vi "Main UI.vi"() -> ()   [LabVIEW 2020, in "App.lvlib" / "MazeUI.lvclass"]
uses:
  MazeUI.lvclass
  build/ppl/maze.lvlibp/Maze/Maze.lvclass
  build/ppl/maze.lvlibp/Mouse/Mouse.lvclass
  build/ppl/maze.lvlibp/Direction.ctl
  <vilib>/Platform/browser.llb/Open URL in Default Browser (string).vi
  build/ppl/maze.lvlibp
  MazeFileIO/MazeFileIO.lvclass
  build/ppl/maze.lvlibp/MazeGen/MazeGen.lvclass
panel:
  in  "Forums":bool
  in  "Configure Mouse":bool
  out "Mouse Name":string="Demo Mouse"
  in  "Run Speed":i32(slide)=100 scale=500.0..0.5
  out "Stepping":bool
  in  "Reset":bool
  in  "Step":bool
  out "Path":picture
  out "Walls":picture
  out "Actions":i32
  out "Mouse":refnum<class "Mouse.lvclass">
  in  "Stop":bool
  out "Running":bool
  out "Maze":refnum<class "Maze.lvclass">
  in  "Save":bool
  in  "Random":bool
  out "Maze":string
  in  "Load Maze":bool
  out "Status":string
  out "Mouse Author":string="Demo Mouse"
  in  "Load Mouse":bool
  in  "Start":bool
  out "Display":picture
  # "Maze Challenge"
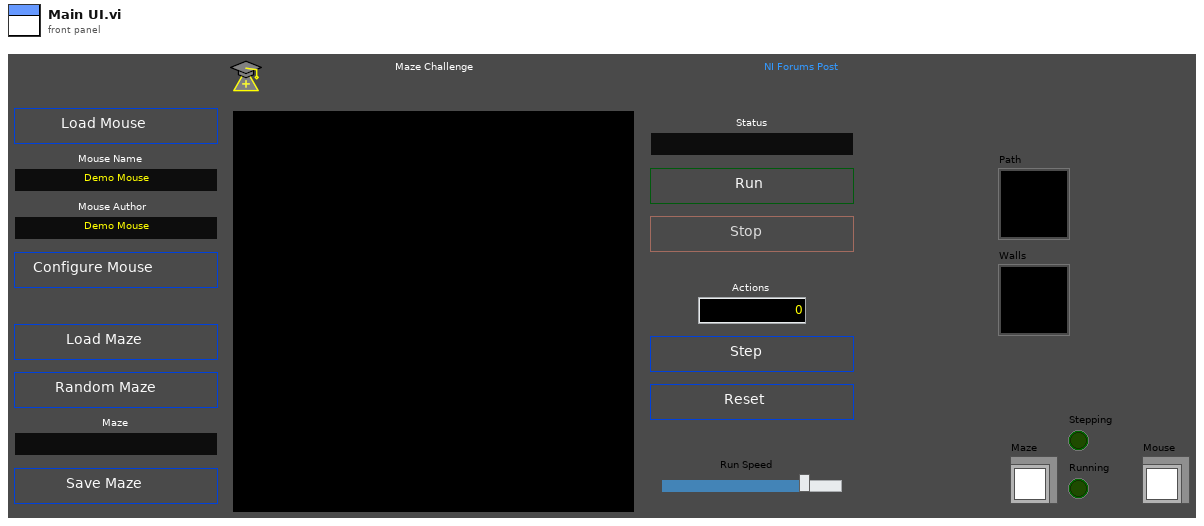
[diagram p1: front panel]
types:
  T1 = enum8{"Enabled", "Disabled", "Disabled and Grayed Out"}
  T2 = typedef "maze.lvlibp/Direction.ctl" = enum8{"East", "North", "West", "South"}
  T3 = typedef "maze.lvlibp/Position.ctl" = cluster{"S":i32, "E":i32}
  T4 = enum32{"invalid app kind", "Development System", "Run Time System", "Student Edition", "Embedded LabVIEW", "Evaluation", "Custom"}
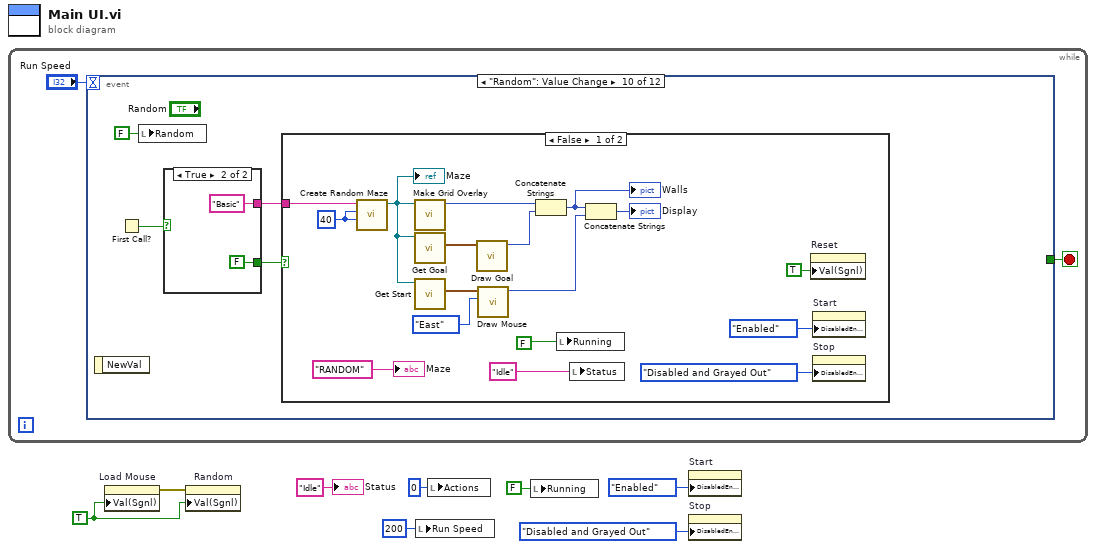
[diagram p0: block diagram]
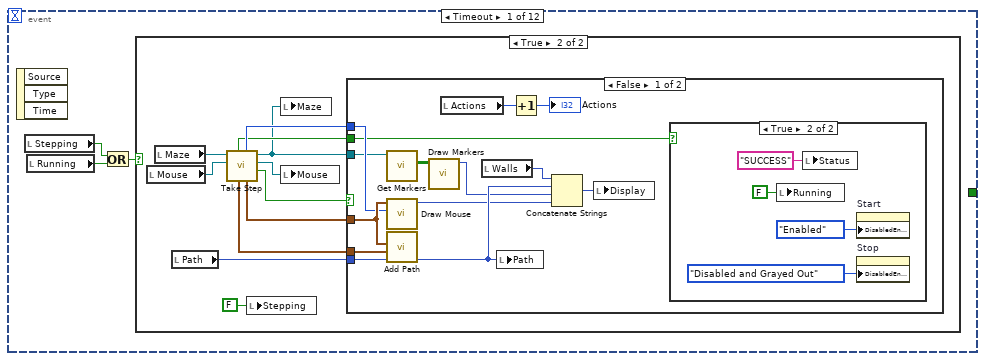
[diagram p2: hidden frame]
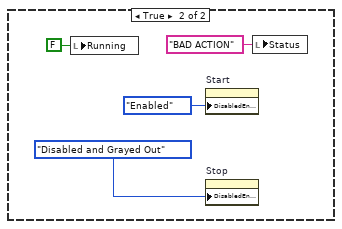
[diagram p5: hidden frame]
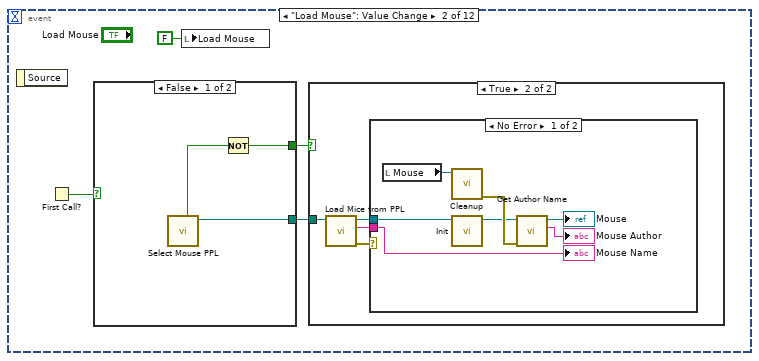
[diagram p6: hidden frame]
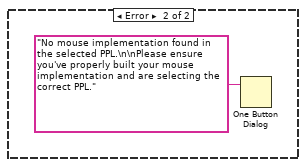
[diagram p8: hidden frame]
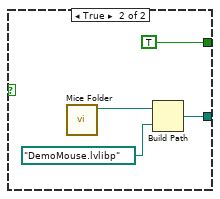
[diagram p9: hidden frame]
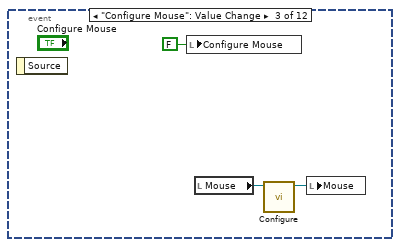
[diagram p10: hidden frame]
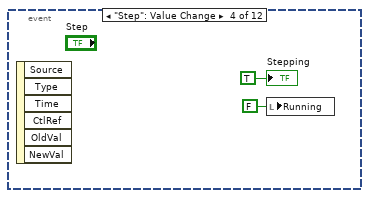
[diagram p11: hidden frame]
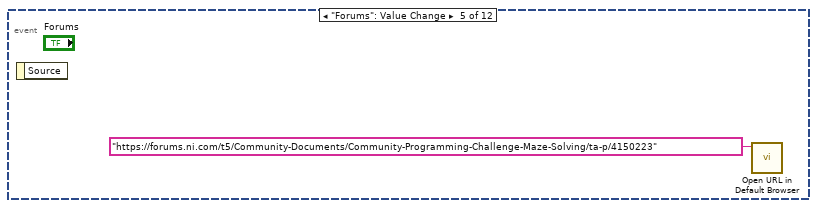
[diagram p12: hidden frame]
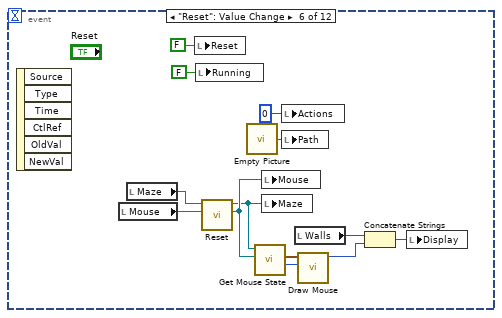
[diagram p13: hidden frame]
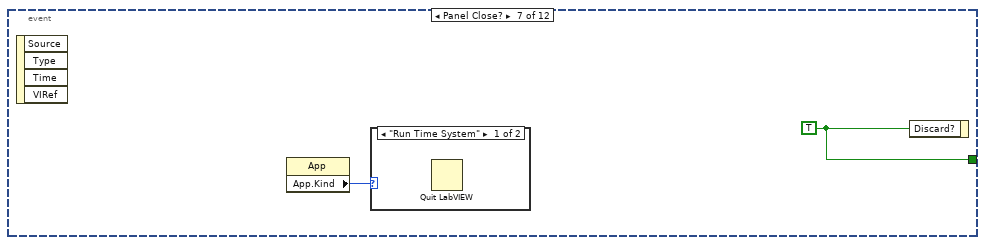
[diagram p14: hidden frame]
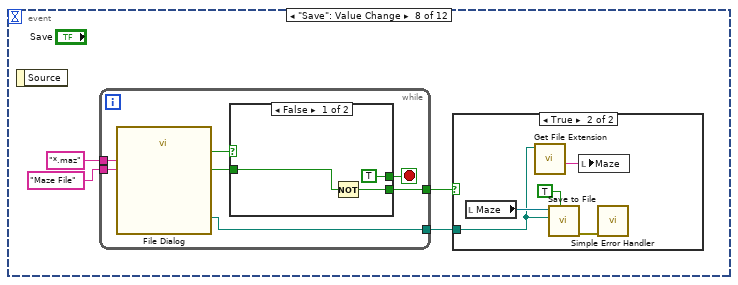
[diagram p16: hidden frame]
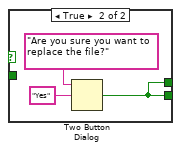
[diagram p18: hidden frame]
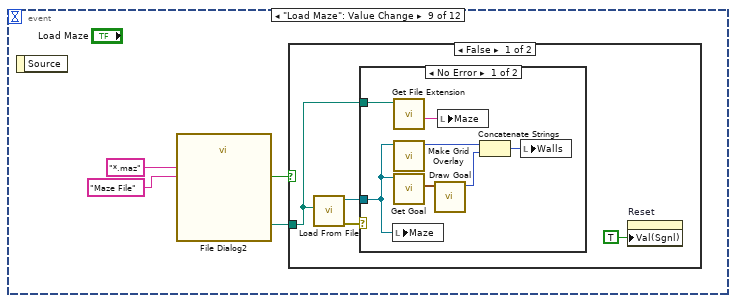
[diagram p19: hidden frame]
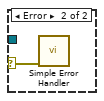
[diagram p20: hidden frame]
diagram:
  w2 = TRUE ("Value (Signaling)")
  n1 = while {
    stop <- w10 stop-if-true
    n2 = event shown="[9] \"Random\": Value Change" {
      selector: _ -> [_ _ _ _ _ _ _ _ _ _ _ _]
      dyn-events: _ -> [_ _ _ _ _ _ _ _ _ _ _ _]
      timeout: "Run Speed" -> [_ _ _ _ _ _ _ _ _ _ _ _]
      tunnel: [_ _ _ _ _ _ w90 _ _ _ _ _] -> w10
      event Timeout {
        n3 = event-data() -> ()  [unwired: 1 in, 3 out]
        n4 = local read "Stepping"() -> (w11:bool)
        n5 = local read "Running"() -> (w13:bool)
        n6 = Or(x=w11, y=w13) -> (x .or. y?=w12:bool)
        n7 = case shown="True" w12 {
          frame False {
          }
          frame True {
            n8 = local read "Mouse"() -> (w16:refnum<class "Mouse.lvclass">)
            n9 = local read "Maze"() -> (w24:refnum<class "Maze.lvclass">)
            n10 = local read "Path"() -> (w19:picture)
            n11 = call "Take Step.vi"("Mouse In"=w16, "Maze in"=w24) -> ("Bad Action?"=w23:bool, "Mouse"=w17:refnum<class "Mouse.lvclass">, "Maze"=w14:refnum<class "Maze.lvclass">, "New Position"=w21:T3, "Direction"=w22:T2, "Old Position"=w20:T3, "Goal?"=w15:bool)  [unwired: 2 in, 1 out]
            n12 = local write "Stepping"(FALSE ("Stepping")) -> ()
            n13 = local write "Maze"(w14) -> ()
            n14 = local write "Mouse"(w17) -> ()
            n15 = case shown="False" w23 {
              tunnel: w22 -> [w30 _]
              tunnel: w21 -> [w31 _]
              tunnel: w20 -> [w37 _]
              tunnel: w19 -> [w38 _]
              tunnel: w15 -> [w29 _]
              tunnel: w14 -> [w27 _]
              frame False {
                n16 = call "Get Markers.vi"("Maze in"=w27) -> ("Markers"=w26:bool[][])  [unwired: 8 in, 2 out]
                n17 = call "Draw Mouse.vi"("Direction"=w30, "Position"=w31) -> ("Picture"=w28:picture)  [unwired: 9 in]
                n18 = call "Add Path.vi"("Path In"=w38, "Old Position"=w37, "New Position"=w31) -> ("Path"=w35:picture)  [unwired: 8 in]
                n19 = call "Draw Markers.vi"("Markers"=w26) -> ("Picture"=w25:picture)  [unwired: 10 in]
                n20 = local read "Actions"() -> (w33:i32)
                n21 = local read "Walls"() -> (w36:picture)
                n22 = local write "Path"(w35) -> ()
                n23 = Increment(x=w33) -> (x+1=→"Actions":i32)
                n24 = Concatenate Strings(w36, w35, w25, w28) -> (w34:picture)
                n25 = local write "Display"(w34) -> ()
                n26 = case shown="True" w29 {
                  frame False {
                  }
                  frame True {
                    n27 = local write "Running"(FALSE ("Running")) -> ()
                    n28 = local write "Status"("SUCCESS" ("Status")) -> ()
                    n29 = property on="Start" class="Bool"("DisabledEnum"=T1."Enabled" ("Disabled")) -> ()  [unwired: 2 in, 2 out]
                    n30 = property on="Stop" class="Bool"("DisabledEnum"=T1."Disabled and Grayed Out" ("Disabled")) -> ()  [unwired: 2 in, 2 out]
                  }
                }
              }
              frame True {
                n31 = local write "Running"(FALSE ("Running")) -> ()
                n32 = property on="Start" class="Bool"("DisabledEnum"=T1."Enabled" ("Disabled")) -> ()  [unwired: 2 in, 2 out]
                n33 = property on="Stop" class="Bool"("DisabledEnum"=T1."Disabled and Grayed Out" ("Disabled")) -> ()  [unwired: 2 in, 2 out]
                n34 = local write "Status"("BAD ACTION" ("Status")) -> ()
              }
            }
          }
        }
      }
      event "Load Mouse": Value Change {
        n35 = event-data() -> ()  [unwired: 1 in, 1 out]
        n36 = First Call?() -> (First Call?: T/F=w49:bool)
        n37 = case shown="False" w49 {
          tunnel: [w63 TRUE] -> w48
          tunnel: [w65 w67] -> w47
          frame False {
            n38 = call "Select Mouse PPL.vi"() -> ("selected path"=w65:path, "cancelled"=w64:bool)  [unwired: 10 in]
            n39 = Not(x=w64) -> (.not. x?=w63:bool)
          }
          frame True {
            n40 = call "Mice Folder.vi"() -> ("Mice Folder"=w66:path)  [unwired: 11 in]
            n41 = Build Path(base path=w66, name or relative path=path "DemoMouse.lvlibp") -> (appended path=w67:path)
          }
        }
        n42 = local write "Load Mouse"(FALSE ("Load Mouse")) -> ()
        n43 = case shown="True" w48 {
          tunnel: w47 -> [_ w54]
          frame False {
          }
          frame True {
            n44 = call "Load Mice from PPL.vi"("Mouse PPL"=w54) -> ("error out"=w51:errorcluster, "Name"=w52:string, "Mouse"=w53:refnum<class "Mouse.lvclass">)  [unwired: 8 in]
            n45 = case shown="No Error" w51 {
              tunnel: w53 -> [w56 _]
              tunnel: w52 -> [w55 _]
              frame No Error {
                n46 = local read "Mouse"() -> (w57:refnum<class "Mouse.lvclass">)
                n47 = call-dynamic "Cleanup.vi"("Mouse in"=w57) -> ("error out"=w61:errorcluster)  [unwired: 10 in]
                n48 = call-dynamic "Init.vi"("Mouse in"=w56) -> ("Mouse out"=w58:refnum<class "Mouse.lvclass">)  [unwired: 9 in, 1 out]
                n49 = call-dynamic "Get Author Name.vi"("error in (no error)"=w61, "Mouse in"=w58) -> ("Author"=→"Mouse Author":string, "Mouse out"=→"Mouse":refnum<class "Mouse.lvclass">)  [unwired: 7 in, 1 out]
                "Mouse Name" <- w55
              }
              frame Error {
                n50 = One Button Dialog(message="No mouse implementation found in the selected PPL.\n\nPlease ensure you've properly built your mouse implementation and are selecting the correct PPL.") -> ()  [unwired: 1 in, 1 out]
              }
            }
          }
        }
      }
      event "Configure Mouse": Value Change {
        n51 = event-data() -> ()  [unwired: 1 in, 1 out]
        n52 = local write "Configure Mouse"(FALSE ("Configure Mouse")) -> ()
        n53 = local read "Mouse"() -> (w71:refnum<class "Mouse.lvclass">)
        n54 = call-dynamic "Configure.vi"("Mouse in"=w71) -> ("Mouse out"=w70:refnum<class "Mouse.lvclass">)  [unwired: 9 in, 1 out]
        n55 = local write "Mouse"(w70) -> ()
      }
      event "Step": Value Change {
        n56 = event-data() -> ()  [unwired: 1 in, 6 out]
        n57 = local write "Running"(FALSE ("Running")) -> ()
        "Stepping" <- TRUE ("Step")
      }
      event "Forums": Value Change {
        n58 = event-data() -> ()  [unwired: 1 in, 1 out]
        n59 = call-poly <vilib>:"Open URL in Default Browser.vi"("URL"="https://forums.ni.com/t5/Community-Documents/Community-Programming-Challenge-Maze-Solving/ta-p/4150223") -> ()  [unwired: 5 in, 2 out]
      }
      event "Reset": Value Change {
        n60 = event-data() -> ()  [unwired: 1 in, 6 out]
        n61 = local read "Mouse"() -> (w77:refnum<class "Mouse.lvclass">)
        n62 = local read "Maze"() -> (w87:refnum<class "Maze.lvclass">)
        n63 = local write "Reset"(FALSE ("Reset")) -> ()
        n64 = local write "Running"(FALSE ("Running")) -> ()
        n65 = call "Reset.vi"("Mouse In"=w77, "Maze in"=w87) -> ("Mouse"=w78:refnum<class "Mouse.lvclass">, "Maze out"=w76:refnum<class "Maze.lvclass">)  [unwired: 7 in, 1 out]
        n66 = call "Empty Picture"() -> ("empty picture"=w88:picture)
        n67 = call "Get Mouse State.vi"("Mouse"=w78, "Maze in"=w76) -> ("Direction"=w80:T2, "Position"=w81:T3)  [unwired: 6 in, 2 out]
        n68 = local write "Mouse"(w78) -> ()
        n69 = local write "Maze"(w76) -> ()
        n70 = local write "Actions"(0 ("Actions")) -> ()
        n71 = local write "Path"(w88) -> ()
        n72 = local read "Walls"() -> (w84:picture)
        n73 = call "Draw Mouse.vi"("Direction"=w80, "Position"=w81) -> ("Picture"=w83:picture)  [unwired: 9 in]
        n74 = Concatenate Strings(w84, w83) -> (w82:picture)
        n75 = local write "Display"(w82) -> ()
      }
      event Panel Close? {
        w90 = TRUE ("Discard?")
        n76 = event-data() -> ()  [unwired: 1 in, 4 out]
        n77 = property class="App"() -> ("App.Kind"=w89:T4)  [unwired: 2 in, 2 out]
        n78 = case shown="\"Run Time System\"" w89 {
          frame "Run Time System" {
            n79 = Quit LabVIEW() -> ()  [unwired: 1 in]
          }
          frame Default {
          }
        }
        n80 = event-data("Discard?"=w90) -> ()  [unwired: 1 in, 1 out]
      }
      event "Save": Value Change {
        n81 = event-data() -> ()  [unwired: 1 in, 1 out]
        n82 = while {
          tunnel: "*.maz" ("pattern (all files)") -> [w106]
          tunnel: "Maze File" ("pattern label") -> [w105]
          tunnel: [w102] -> w91
          tunnel: [w100] -> w92
          stop <- w101 stop-if-true
          n83 = call "File Dialog"("pattern (all files)"=w106, "pattern label"=w105) -> ("selected path"=w100:path, "exists"=w104:bool, "cancelled"=w103:bool)  [unwired: 10 in, 1 out]
          n84 = case shown="False" w104 {
            tunnel: w103 -> [w108 _]
            tunnel: [w109 w110] -> w102
            tunnel: [TRUE ("T button?") w110] -> w101
            frame False {
              n85 = Not(x=w108) -> (.not. x?=w109:bool)
            }
            frame True {
              n86 = Two Button Dialog(message="Are you sure you want to replace the file?", 2:"Yes" ("T button name (\"OK\")")) -> (T button?=w110:bool)  [unwired: 1 in]
            }
          }
        }
        n87 = case shown="True" w91 {
          tunnel: w92 -> [_ w96]
          frame False {
          }
          frame True {
            n88 = local read "Maze"() -> (w99:refnum<class "Maze.lvclass">)
            n89 = call <vilib>:"Get File Extension.vi"("file"=w96) -> ("filename without extension"=w95:string)  [unwired: 6 in, 4 out]
            n90 = call "Save to File.vi"("Replace if Exists? (F)"=TRUE, "Maze File Path (*.maz)"=w96, "Maze In"=w99) -> ("error out"=w97:errorcluster)  [unwired: 7 in, 1 out]
            n91 = local write "Maze"(w95) -> ()
            n92 = call <vilib>:"Simple Error Handler.vi"("error in (no error)"=w97) -> ()  [unwired: 4 in, 5 out]
          }
        }
      }
      event "Load Maze": Value Change {
        n93 = event-data() -> ()  [unwired: 1 in, 1 out]
        n94 = call "File Dialog2"("pattern (all files)"="*.maz", "pattern label"="Maze File") -> ("selected path"=w116:path, "cancelled"=w113:bool)  [unwired: 10 in, 2 out]
        n95 = case shown="False" w113 {
          tunnel: w116 -> [w117 _]
          frame False {
            n96 = call "Load From File.vi"("Maze File Path (*.maz)"=w117) -> ("error out"=w118:errorcluster, "Maze"=w120:refnum<class "Maze.lvclass">)  [unwired: 9 in]
            n97 = case shown="No Error" w118 {
              selector: w118 -> [_ w128]
              tunnel: w120 -> [w123 _]
              tunnel: w117 -> [w122 _]
              frame No Error {
                n98 = local write "Maze"(w123) -> ()
                n99 = call <vilib>:"Get File Extension.vi"("file"=w122) -> ("filename without extension"=w121:string)  [unwired: 6 in, 4 out]
                n100 = call "Make Grid Overlay.vi"("Maze"=w123) -> ("Picture"=w126:picture)  [unwired: 10 in]
                n101 = call "Get Goal.vi"("Maze in"=w123) -> ("Goal"=w125:T3)  [unwired: 8 in, 2 out]
                n102 = call "Draw Goal.vi"("Position"=w125) -> ("Picture"=w124:picture)  [unwired: 10 in]
                n103 = local write "Maze"(w121) -> ()
                n104 = Concatenate Strings(w126, w124) -> (w127:picture)
                n105 = local write "Walls"(w127) -> ()
              }
              frame Error {
                n106 = call <vilib>:"Simple Error Handler.vi"("error in (no error)"=w128) -> ()  [unwired: 4 in, 5 out]
              }
            }
            n107 = property on="Reset" class="Bool (strict)"("Val(Sgnl)"=TRUE ("Value (Signaling)")) -> ()  [unwired: 2 in, 2 out]
          }
          frame True {
          }
        }
      }
      event "Random": Value Change {
        n108 = event-data() -> ()  [unwired: 1 in, 1 out]
        n109 = First Call?() -> (First Call?: T/F=w129:bool)
        n110 = local write "Random"(FALSE ("Random")) -> ()
        n111 = case shown="True" w129 {
          tunnel: [w134 "Basic" ("Selected Level")] -> w131
          tunnel: [w133 FALSE ("Cancelled?")] -> w130
          frame False {
            n112 = call "Select Level UI.vi"() -> ("Cancelled?"=w133:bool, "Selected Level"=w134:string)  [unwired: 10 in]
          }
          frame True {
          }
        }
        n113 = case shown="False" w130 {
          tunnel: w131 -> [w137 _]
          frame False {
            w138 = 40 ("Height")
            n114 = call "Create Random Maze.vi"("Height (40)"=w138, "Width (40)"=w138, "Maze Level"=w137) -> ("Maze"=w139:refnum<class "Maze.lvclass">)  [unwired: 7 in, 1 out]
            "Maze" <- w139
            n115 = call "Make Grid Overlay.vi"("Maze"=w139) -> ("Picture"=w153:picture)  [unwired: 10 in]
            n116 = call "Get Goal.vi"("Maze in"=w139) -> ("Goal"=w150:T3)  [unwired: 8 in, 2 out]
            n117 = call "Get Start.vi"("Maze in"=w139) -> ("Start"=w152:T3)  [unwired: 8 in, 2 out]
            n118 = call "Draw Goal.vi"("Position"=w150) -> ("Picture"=w149:picture)  [unwired: 10 in]
            n119 = call "Draw Mouse.vi"("Direction"=Direction."East", "Position"=w152) -> ("Picture"=w145:picture)  [unwired: 9 in]
            n120 = Concatenate Strings(w153, w149) -> (w147:picture)
            "Walls" <- w147
            n121 = local write "Running"(FALSE ("Running")) -> ()
            n122 = local write "Status"("Idle" ("Status")) -> ()
            n123 = Concatenate Strings(w147, w145) -> (→"Display":picture)
            n124 = property on="Reset" class="Bool (strict)"("Val(Sgnl)"=TRUE ("Value (Signaling)")) -> ()  [unwired: 2 in, 2 out]
            n125 = property on="Start" class="Bool"("DisabledEnum"=T1."Enabled" ("Disabled")) -> ()  [unwired: 2 in, 2 out]
            n126 = property on="Stop" class="Bool"("DisabledEnum"=T1."Disabled and Grayed Out" ("Disabled")) -> ()  [unwired: 2 in, 2 out]
            "Maze" <- "RANDOM" ("Maze")
          }
          frame True {
          }
        }
      }
      event "Start": Value Change {
        n127 = event-data() -> ()  [unwired: 1 in, 1 out]
        n128 = local read "Mouse"() -> (w157:refnum<class "Mouse.lvclass">)
        n129 = local read "Maze"() -> (w158:refnum<class "Maze.lvclass">)
        n130 = call "Empty Picture"() -> ("empty picture"=→"Path":picture)
        n131 = call "Reset.vi"("Mouse In"=w157, "Maze in"=w158) -> ("Mouse"=w156:refnum<class "Mouse.lvclass">, "Maze out"=w154:refnum<class "Maze.lvclass">)  [unwired: 7 in, 1 out]
        n132 = local write "Status"("Running" ("Status")) -> ()
        n133 = call-dynamic "Start.vi"("Mouse in"=w156) -> ("Mouse out"=w155:refnum<class "Mouse.lvclass">)  [unwired: 9 in, 1 out]
        n134 = local write "Maze"(w154) -> ()
        n135 = local write "Actions"(0 ("Actions")) -> ()
        n136 = local write "Mouse"(w155) -> ()
        n137 = property on="Start" class="Bool"("DisabledEnum"=T1."Disabled and Grayed Out" ("Disabled")) -> ()  [unwired: 2 in, 2 out]
        n138 = property on="Stop" class="Bool"("DisabledEnum"=T1."Enabled" ("Disabled")) -> ()  [unwired: 2 in, 2 out]
        "Running" <- TRUE ("Running")
      }
      event "Stop": Value Change {
        n139 = event-data() -> ()  [unwired: 1 in, 6 out]
        n140 = local write "Running"(FALSE ("Running")) -> ()
        n141 = local write "Status"("Idle" ("Status")) -> ()
        n142 = property on="Start" class="Bool"("DisabledEnum"=T1."Enabled" ("Disabled")) -> ()  [unwired: 2 in, 2 out]
        n143 = property on="Stop" class="Bool"("DisabledEnum"=T1."Disabled and Grayed Out" ("Disabled")) -> ()  [unwired: 2 in, 2 out]
      }
    }
  }
  n144 = property on="Load Mouse" class="Bool (strict)"("Val(Sgnl)"=w2) -> (error out=w1:errorcluster)  [unwired: 2 in, 1 out]
  n145 = property on="Random" class="Bool (strict)"(error in=w1, "Val(Sgnl)"=w2) -> ()  [unwired: 1 in, 2 out]
  n146 = local write "Run Speed"(200 ("Run Speed")) -> ()
  n147 = local write "Actions"(0 ("Actions")) -> ()
  n148 = local write "Running"(FALSE ("Running")) -> ()
  n149 = property on="Start" class="Bool"("DisabledEnum"=T1."Enabled" ("Disabled")) -> ()  [unwired: 2 in, 2 out]
  n150 = property on="Stop" class="Bool"("DisabledEnum"=T1."Disabled and Grayed Out" ("Disabled")) -> ()  [unwired: 2 in, 2 out]
  "Status" <- "Idle" ("Status")
